vi "LogEngine.LogFile.Write.vi"(8 "error in (no error)":errorcluster, 10 "Data":T1[](array[typedef]), 11 "Byte Stream File in":refnum<file>) -> (0 "error out":errorcluster, 3 "Byte Stream File out":refnum<file>)   [LabVIEW 2025, in "XNET Bus Monitor Client.lvlib"]
uses:
  XNET Bus Monitor Client.lvlib
  bus_monitor_client/RPC Messages/ni_bus_monitor_api_Frame.ctl
  bus_monitor_client/bus_monitor_client.lvlib
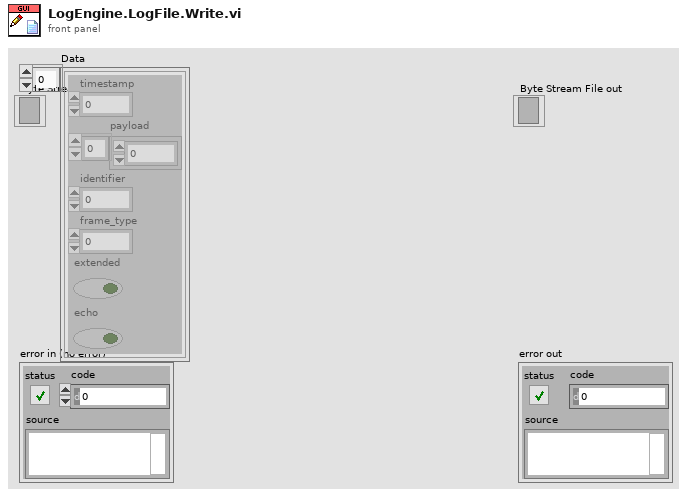
[diagram p1: front panel]
types:
  T1 = typedef "bus_monitor_client.lvlib/ni_bus_monitor_api_Frame.ctl" = cluster{"timestamp":dbl, "payload":u8[], "identifier":u32, "frame_type":u32, "extended":bool, "echo":bool}
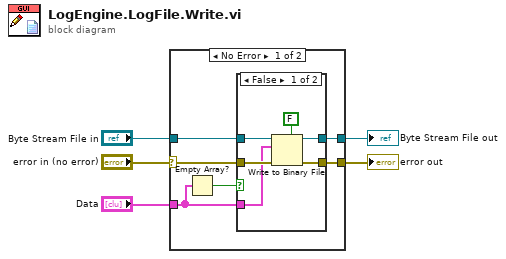
[diagram p0: block diagram]
diagram:
  n1 = case shown="No Error" "error in (no error)" {
    selector: "error in (no error)" -> [w8 w21]
    tunnel: [w11 w21] -> w5
    tunnel: [w10 w20] -> w4
    tunnel: "Byte Stream File in" -> [w9 w20]
    tunnel: "Data" -> [w7 _]
    frame No Error {
      n2 = Empty Array?(array=w7) -> (empty?=w6:bool)
      n3 = case shown="False" w6 {
        tunnel: [w17 w19] -> w11
        tunnel: [w16 w18] -> w10
        tunnel: w9 -> [w15 w18]
        tunnel: w8 -> [w14 w19]
        tunnel: w7 -> [w13 _]
        frame False {
          n4 = Write to Binary File(file (use dialog)=w15, data=w13, error in=w14, 5:FALSE ("prepend array or string size? (T)")) -> (refnum out=w16:refnum<file>, error out=w17:errorcluster)  [unwired: 2 in, 1 out]
        }
        frame True {
        }
      }
    }
    frame Error {
    }
  }
  "error out" <- w5
  "Byte Stream File out" <- w4
